vi "Write Main VI.vi"(8 "error in (no error)":errorcluster, 10 "Main VI":refnum<vi>, 11 "Tax_calculation in":refnum<class "Tax_calculation.lvclass">) -> (0 "error out":errorcluster, 3 "Tax_calculation out":refnum<class "Tax_calculation.lvclass">)   [LabVIEW 2016, in "Tax_calculation.lvclass"]
uses:
  Tax_calculation.lvclass
  Tax_calculation.lvclass/Tax_calculation.ctl
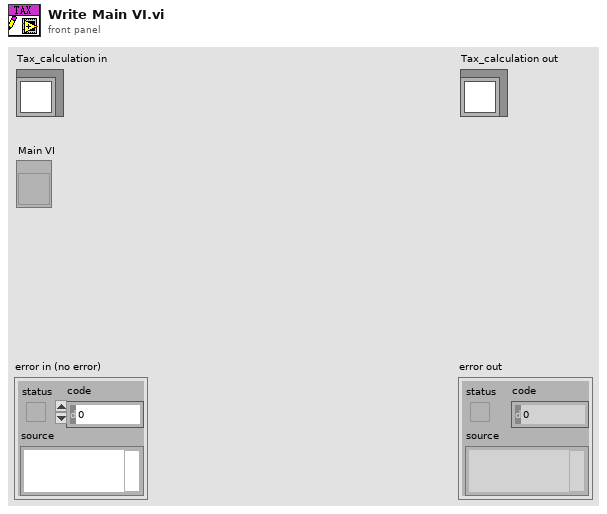
[diagram p1: front panel]
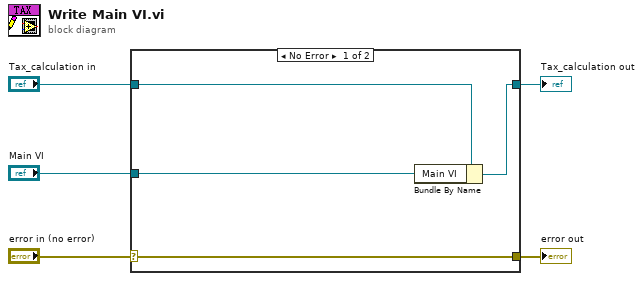
[diagram p0: block diagram]
diagram:
  n1 = case shown="No Error" "error in (no error)" {
    selector: "error in (no error)" -> [w9 w10]
    tunnel: [w9 w10] -> w4
    tunnel: [w7 w11] -> w2
    tunnel: "Tax_calculation in" -> [w8 w11]
    tunnel: "Main VI" -> [w6 _]
    frame No Error {
      n2 = Bundle By Name(cluster=w8, "Main VI"=w6) -> (w7:refnum<class "Tax_calculation.lvclass">)
    }
    frame Error {
    }
  }
  "error out" <- w4
  "Tax_calculation out" <- w2
